vi "Get Employee Salary Info Names and Types Array.vi"(8 "error in (no error)":errorcluster caption="错误输入（无错误）", 11 "Employee 输入":refnum<class "Employee.lvclass"> caption="DNL_LabVIEW Object in") -> (0 "error out":errorcluster caption="错误输出", 1 "Colomn Types":variant[](array[variant]), 2 "Column Names":string[](array[string]), 3 "Employee 输出":refnum<class "Employee.lvclass"> caption="DNL_LabVIEW Object out")   [LabVIEW 2012, in "Employee.lvclass"]
uses:
  Employee.lvclass
  Custom Def/Salary Info.ctl
panel:
  in  "Salary Info":T1
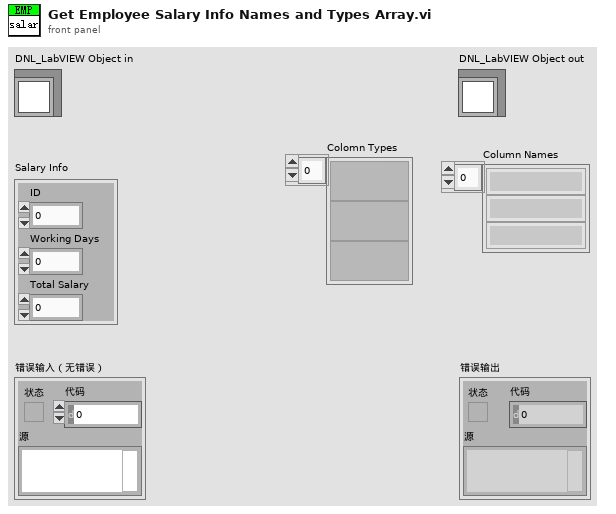
[diagram p1: front panel]
types:
  T1 = typedef "Salary Info.ctl" = cluster{"ID":u16, "Working Days":dbl, "Total Salary":dbl}
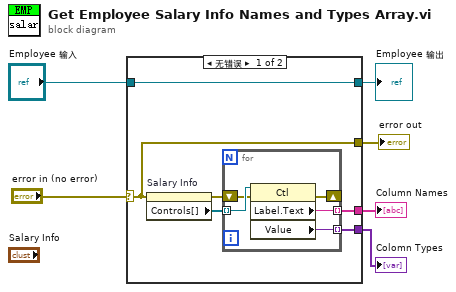
[diagram p0: block diagram]
diagram:
  n1 = case shown="无错误" "error in (no error)" {
    selector: "error in (no error)" -> [w11 w19]
    tunnel: [w11 w19] -> w5
    tunnel: [w12 w18] -> w3
    tunnel: "Employee 输入" -> [w12 w18]
    tunnel: [w8 _] -> w2
    tunnel: [w7 _] -> w1
    frame No Error {
      n2 = property on="Salary Info" class="Clust (严格)"(error in=w11) -> (error out=w10:errorcluster, "Controls[]"=w9:refnum<vi>[])  [unwired: 1 in, 1 out]
      n3 = for {
        tunnel: w9 -> [w17] mode=indexing
        tunnel: [w16] -> w8 mode=indexing
        tunnel: [w15] -> w7 mode=indexing
        shift-right: [w13] -> _
        shift-left: w10 -> [w14]
        n4 = property class="Ctl"(reference=w17, error in=w14) -> (error out=w13:errorcluster, "Label.Text"=w16:string, "Value"=w15:variant)  [unwired: 1 out]
      }
    }
    frame Error {
    }
  }
  "error out" <- w5
  "Employee 输出" <- w3
  "Colomn Types" <- w1
  "Column Names" <- w2
